vi "MU Get Version String.vi"(8 "error in (no error)":errorcluster) -> (0 "error out (no error)":errorcluster, 3 "versionString":string)   [LabVIEW 2017, in "MU_3SL_interface.lvlib"]
uses:
  MU_3SL_interface.lvlib
  lib/MU_3SL_interface.dll
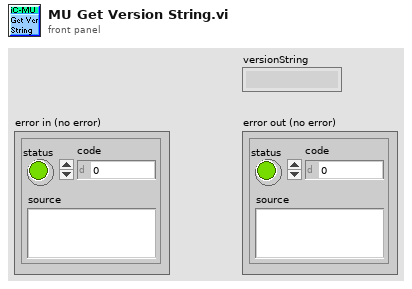
[diagram p1: front panel]
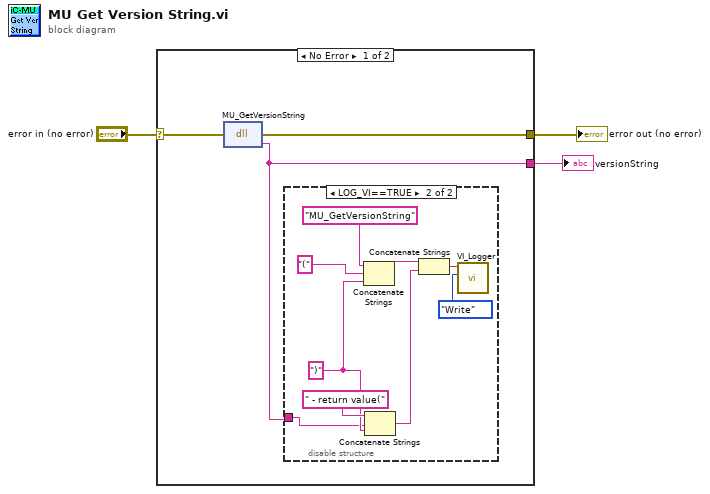
[diagram p0: block diagram]
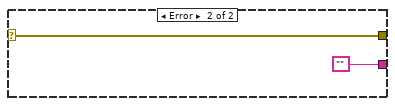
[diagram p3: hidden frame]
diagram:
  n1 = case shown="No Error" "error in (no error)" {
    selector: "error in (no error)" -> [w6 w17]
    tunnel: [w5 w17] -> w3
    tunnel: [w4 ""] -> w1
    frame No Error {
      n2 = dll-call lib="C:/Users/bes/AppData/Roaming/work/mu_9so/icsubmodules/soft_mu_3sl_master/lv_interface/lib/MU_3SL_interface**.*" fn="MU_GetVersionString"(error in=w6) -> (error out=w5:errorcluster, "return type"=w4:string)  [unwired: 2 in, 1 out]
      n3 = disable-structure shown="LOG_VI==TRUE" {
        disable-tunnel: w4 -> [_ w7]
        frame condition #0 {
        }
        frame condition #1 (active) {
          w8 = ")" ("string")
          n4 = Concatenate Strings("MU_GetVersionString" ("Info in"), "(" ("string"), w8) -> (w13:string)
          n5 = Concatenate Strings(" - return value(" ("string"), w7, w8) -> (w12:string)
          n6 = Concatenate Strings(w13, w12) -> (w11:string)
          n7 = call "VI_Logger.vi"("Action (Read)"=enum16{"Write", "Read"}."Write", "Info in"=w11) -> ()  [unwired: 8 in, 2 out]
        }
      }
    }
    frame Error {
    }
  }
  "error out (no error)" <- w3
  "versionString" <- w1
